vi "Read FpgaRef5782.vi"(8 "error in (no error)":errorcluster, 11 "Scope5761 in":refnum<class "Scope5782_six_channel.lvclass">) -> (0 "error out":errorcluster, 2 "FpgaRef5785.lvclass":refnum<class "FpgaRef5785.lvclass">, 3 "Scope5761 out":refnum<class "Scope5782_six_channel.lvclass">)   [LabVIEW 2018, in "Scope5782_six_channel.lvclass"]
uses:
  Scope5782_six_channel.lvclass
  FpgaRef/FpgaRef5785/FpgaRef5785.lvclass
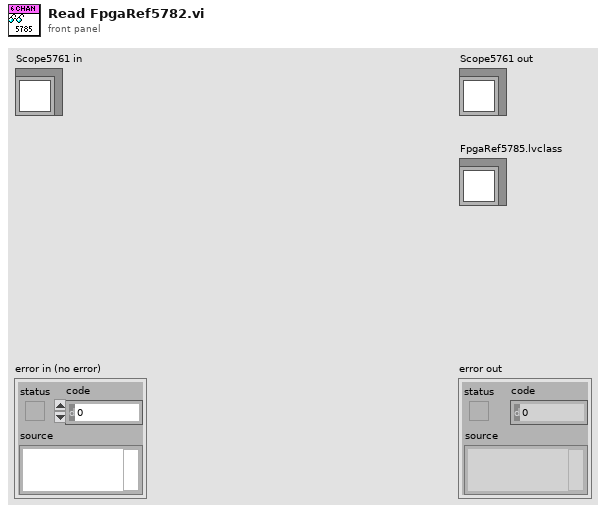
[diagram p1: front panel]
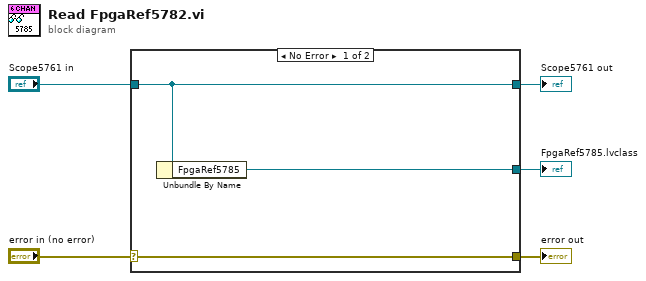
[diagram p0: block diagram]
diagram:
  n1 = case shown="No Error" "error in (no error)" {
    selector: "error in (no error)" -> [w8 w9]
    tunnel: [w8 w9] -> w4
    tunnel: [w7 w10] -> w2
    tunnel: "Scope5761 in" -> [w7 w10]
    tunnel: [w6 _] -> w1
    frame No Error {
      n2 = Unbundle By Name(w7) -> ("FpgaRef5785"=w6:refnum<class "FpgaRef5785.lvclass">)
    }
    frame Error {
    }
  }
  "error out" <- w4
  "Scope5761 out" <- w2
  "FpgaRef5785.lvclass" <- w1
